vi "ROI group-Obtain X-Axis max min.vi"(9 "ROI group data":T1, 11 "Max min-shift in":cluster{"Max":dbl, "Min":dbl}) -> (3 "Max min out":cluster{dbl, dbl})   [LabVIEW 2020]
uses:
  xcontrol/Interface VIs/Interface typedefs/Interface-Data format definition.ctl
  xcontrol/Typedefs/Xctl-XY data type definition.ctl
  xcontrol/Typedefs/Xctrl-ROI type enum.ctl
  xcontrol/XGrapher.xctl
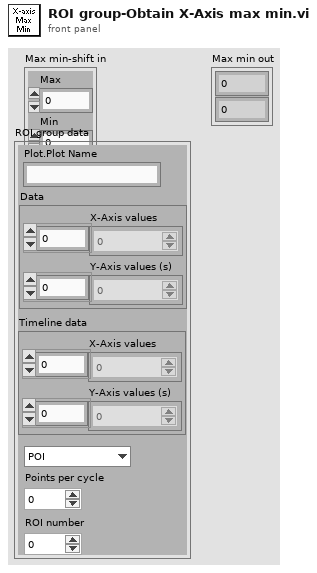
[diagram p1: front panel]
types:
  T1 = typedef "Interface-Data format definition.ctl" = cluster{"Plot.Plot Name":string, "Data":T2, "Timeline data":T2, "Type":T3, "Points per cycle":u16, "ROI number":u16}
  T2 = typedef "XGrapher.xctl/Xctl-XY data type definition.ctl" = cluster{"X-Axis values":sgl[], "Y-Axis values (s)":sgl[]}
  T3 = typedef "Xctrl-ROI type enum.ctl" = enum16{"POI", "Mini-scan", "Group"}
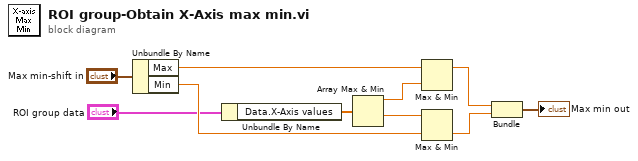
[diagram p0: block diagram]
diagram:
  n1 = Unbundle By Name("Max min-shift in") -> ("Max"=w5:dbl, "Min"=w9:dbl)
  n2 = Unbundle By Name("ROI group data") -> ("Data.X-Axis values"=w2:sgl[])
  n3 = Array Max & Min(array=w2) -> (max value=w6:sgl, min value=w8:sgl)  [unwired: 2 out]
  n4 = Max & Min(x=w5, y=w6) -> (max(x,y)=w7:dbl)  [unwired: 1 out]
  n5 = Max & Min(x=w8, y=w9) -> (min(x,y)=w10:dbl)  [unwired: 1 out]
  n6 = Bundle(w7, w10) -> (→"Max min out":cluster{dbl, dbl})  [unwired: 1 in]
